vi "ListAllValue.vi"(8 "Language":u32, 9 "值表数组":string[][](array[string])) -> (3 "所有信号的值表":string(tree))   [LabVIEW 2015]
panel:
  out "txtTitle":string
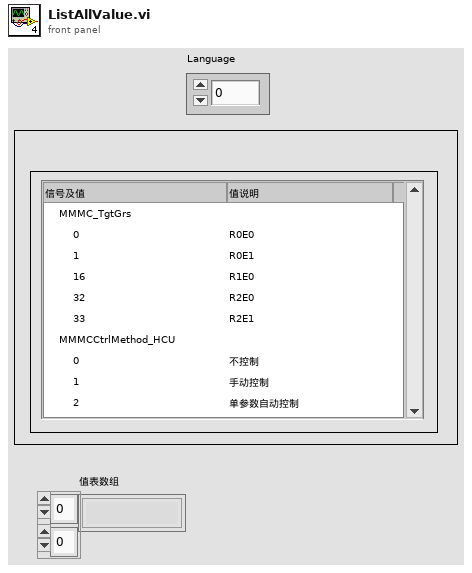
[diagram p1: front panel]
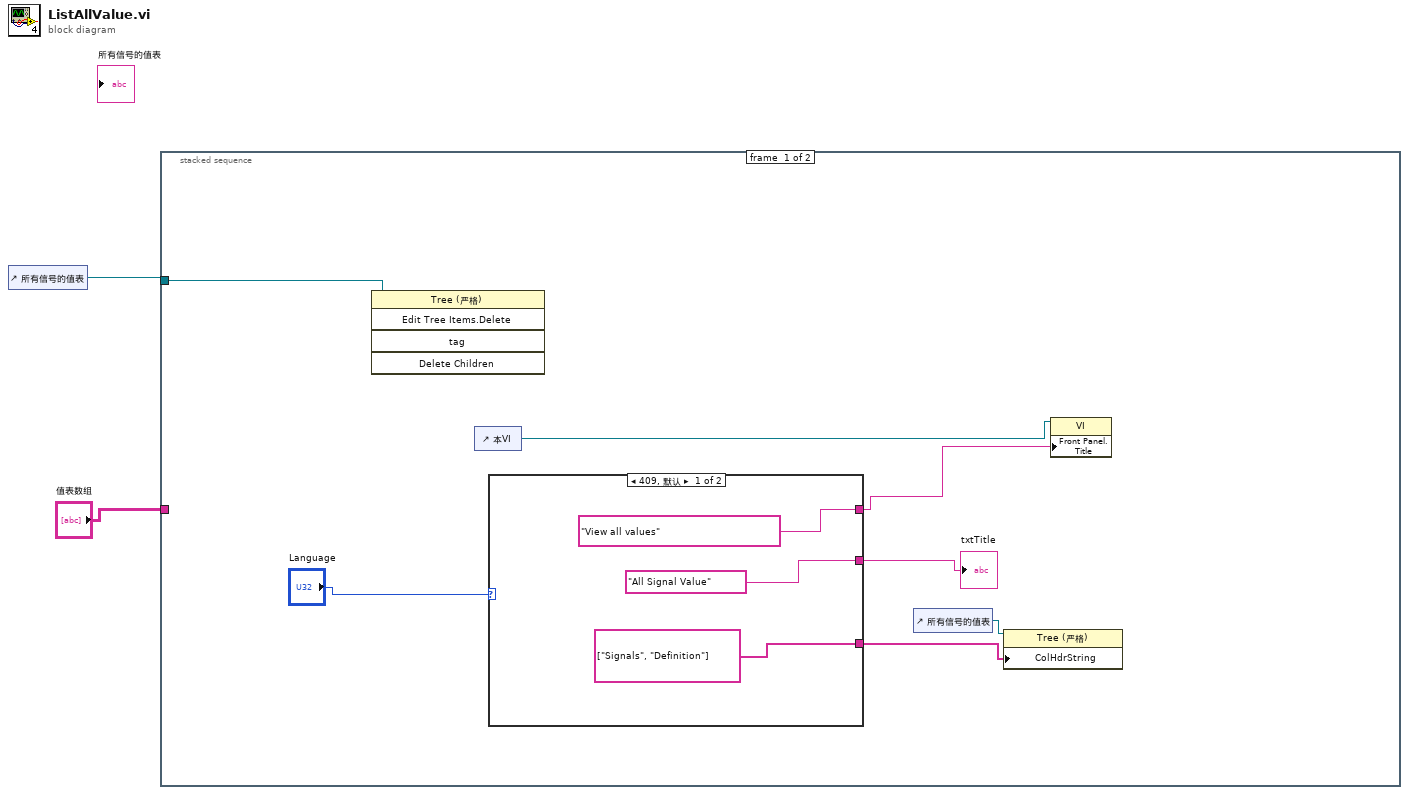
[diagram p0: block diagram]
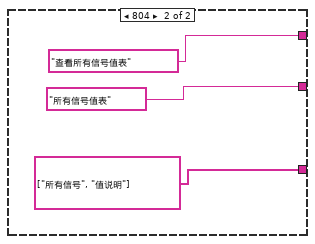
[diagram p2: hidden frame]
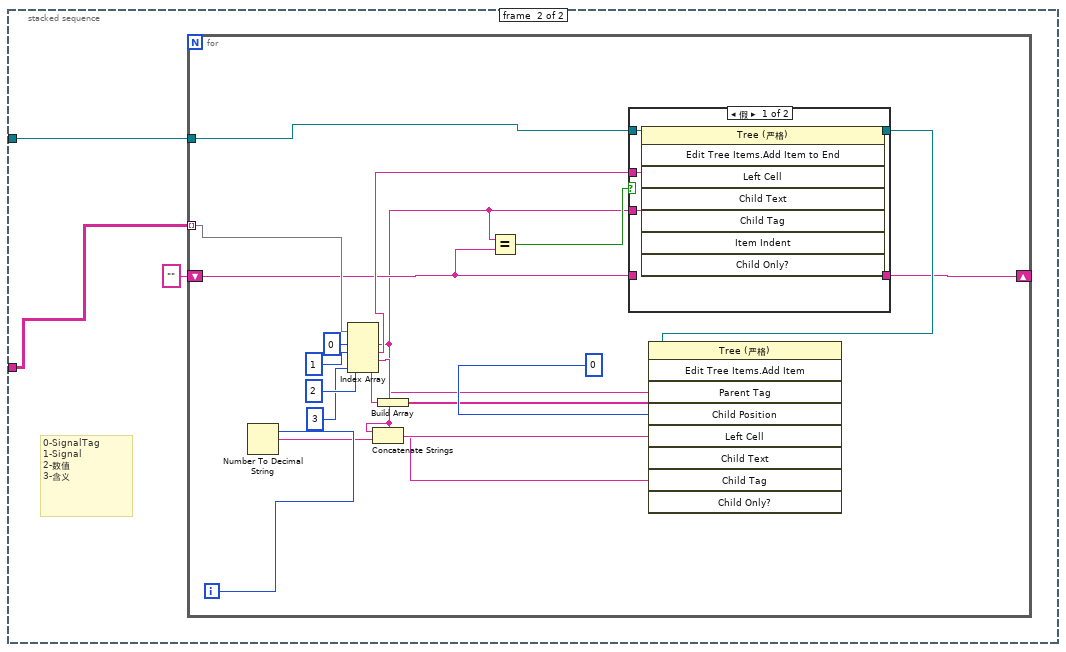
[diagram p3: hidden frame]
diagram:
  n1 = control-ref of="所有信号的值表"() -> (w2:refnum<vi>)
  n2 = stacked-sequence {
    tunnel: w2 -> [w9 w18]
    tunnel: "值表数组" -> [_ w17]
    frame #0 {
      n3 = invoke class="Tree (严格)" method="Edit Tree Items.Delete"(reference=w9) -> ()  [unwired: 4 in, 5 out]
      n4 = control-ref of="本VI"() -> (w6:refnum<vi>)
      n5 = case shown="409, 默认" "Language" {
        tunnel: ["View all values" "查看所有信号值表"] -> w5
        tunnel: [string[] ["Signals", "Definition"] string[] ["所有信号", "值说明"]] -> w3
        tunnel: ["All Signal Value" "所有信号值表"] -> w8
        frame 409, Default {
        }
        frame 804 {
        }
      }
      "txtTitle" <- w8
      n6 = control-ref of="所有信号的值表"() -> (w4:refnum<vi>)
      n7 = property class="Tree (严格)"(reference=w4, "ColHdrString"=w3) -> ()  [unwired: 1 in, 2 out]
      n8 = property class="VI"(reference=w6, "Front Panel.Title"=w5) -> ()  [unwired: 1 in, 2 out]
    }
    frame #1 {
      # "0-SignalTag\n1-Signal\n2-数值\n3-含义"
      n9 = for {
        tunnel: w18 -> [w37]
        tunnel: w17 -> [w36] mode=indexing
        shift-right: [w22] -> _
        shift-left: "" ("String") -> [w20]
        i -> [w35]
        n10 = Number To Decimal String(number=w35) -> (decimal integer string=w34:string)  [unwired: 1 in]
        n11 = Index Array(array=w36, index #1=0 ("索引"), index #2=1 ("索引"), index #3=2 ("索引"), index #4=3 ("索引")) -> (element #1=w19:string, element #2=w29:string, element #3=w25:string, element #4=w26:string)
        n12 = Concatenate Strings(w25, w34) -> (w24:string)
        n13 = Build Array(w26) -> (w27:string[])
        n14 = Equal?(x=w19, y=w20) -> (x = y?=w21:bool)
        n15 = case shown="假" w21 {
          tunnel: w29 -> [w41 _]
          tunnel: w37 -> [w40 w43]
          tunnel: w19 -> [w38 _]
          tunnel: [w39 w43] -> w23
          tunnel: [w38 w42] -> w22
          tunnel: w20 -> [_ w42]
          frame False {
            n16 = invoke class="Tree (严格)" method="Edit Tree Items.Add Item to End"(reference=w40, "Left Cell"=w41, "Child Tag"=w38) -> (reference out=w39:refnum<vi>)  [unwired: 5 in, 7 out]
          }
          frame True {
          }
        }
        n17 = invoke class="Tree (严格)" method="Edit Tree Items.Add Item"(reference=w23, "Parent Tag"=w19, "Child Position"=0 ("子项位置"), "Left Cell"=w25, "Child Text"=w27, "Child Tag"=w24) -> ()  [unwired: 3 in, 9 out]
      }
    }
  }
